vi "SubVi.Sorting an ini file using a cluster.vi"(1 "Array in":T1(array[cluster]), 2 "Cluster structure":T2) -> (0 "Array out":T1(array[cluster]))   [LabVIEW 2015]
doc: "Sorting an ini file using a cluster"
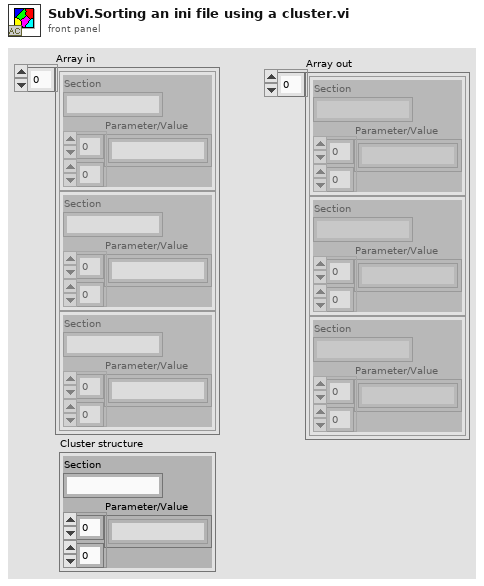
[diagram p1: front panel]
types:
  T1 = cluster{"Section":string, "Parameter/Value":string[][]}[]
  T2 = cluster{"Section":string, "Parameter/Value":string[][]}
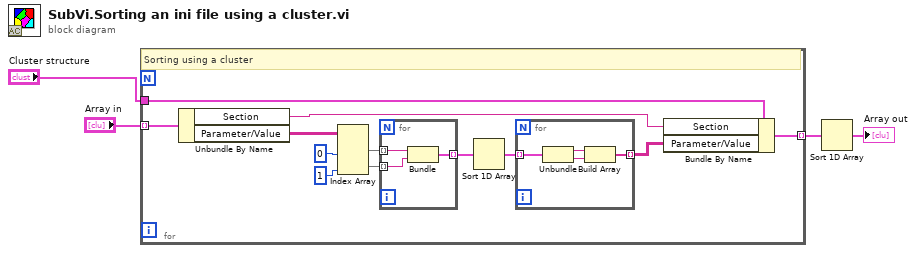
[diagram p0: block diagram]
diagram:
  n1 = for {
    tunnel: "Array in" -> [w16] mode=indexing
    tunnel: "Cluster structure" -> [w15]
    tunnel: [w14] -> w1 mode=indexing
    # "Sorting using a cluster"
    n2 = Unbundle By Name(w16) -> ("Section"=w13:string, "Parameter/Value"=w6:string[][])
    n3 = Index Array(array=w6, index (col) #1=0, index (col) #2=1) -> (element #1=w10:string[], element #2=w9:string[])  [unwired: 2 in]
    n4 = for {
      tunnel: w10 -> [w23] mode=indexing
      tunnel: w9 -> [w22] mode=indexing
      tunnel: [w21] -> w8 mode=indexing
      n5 = Bundle("String"=w23, "String"=w22) -> (w21:cluster{"String":string, "String":string})  [unwired: 1 in]
    }
    n6 = Sort 1D Array(array=w8) -> (sorted array=w7:cluster{"String":string, "String":string}[])
    n7 = for {
      tunnel: w7 -> [w20] mode=indexing
      tunnel: [w17] -> w5 mode=indexing
      n8 = Unbundle(w20) -> ("String"=w19:string, "String"=w18:string)
      n9 = Build Array(w19, w18) -> (w17:string[])
    }
    n10 = Bundle By Name(cluster=w15, "Section"=w13, "Parameter/Value"=w5) -> (w14:T2)
  }
  n11 = Sort 1D Array(array=w1) -> (sorted array=→"Array out":T1)
